vi "ABB Report NoLoad.vi"(10 "Report in":string) -> (2 "Report out":string, 3 "jpg  path":path)   [LabVIEW 2017]
uses:
  ABB global.vi
panel:
  out "Separation of losses":cluster{dbl[], "Best Linear Fit":dbl[]}[](graph)
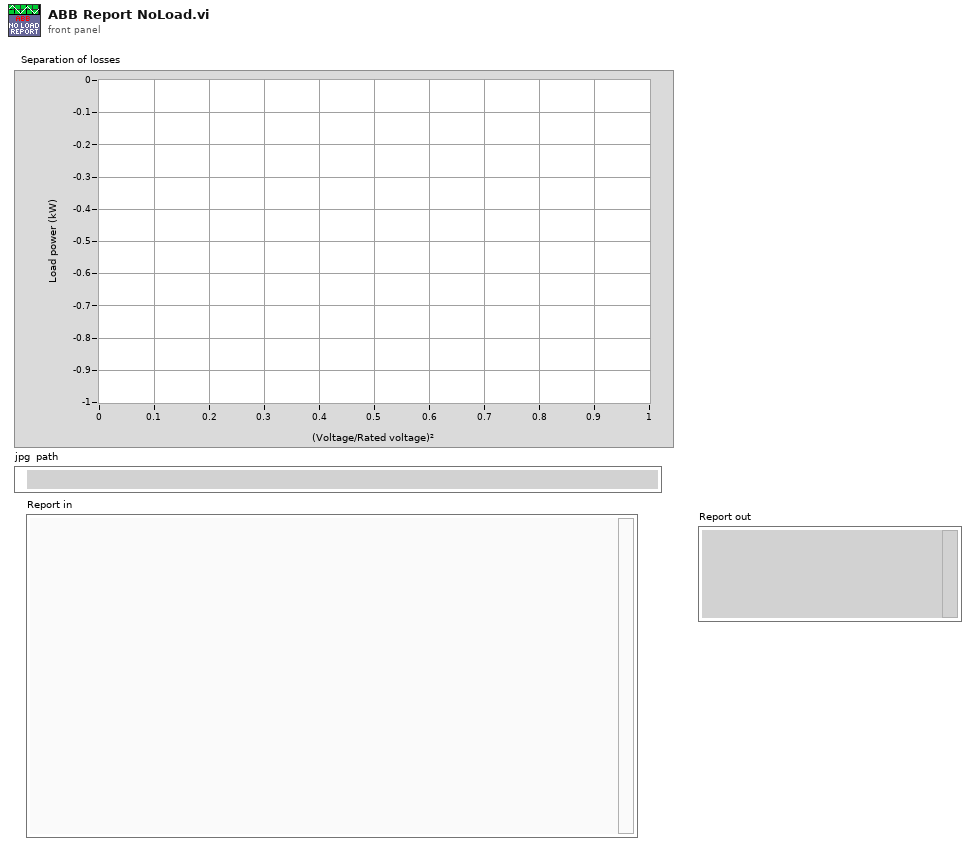
[diagram p1: front panel]
types:
  T1 = cluster{"PCu":dbl, "Pmech":dbl, "PFe":dbl, "Ptot":dbl, "Ambient":dbl, "I1":dbl, "I2":dbl, "I3":dbl, "Wdg Temp":dbl}
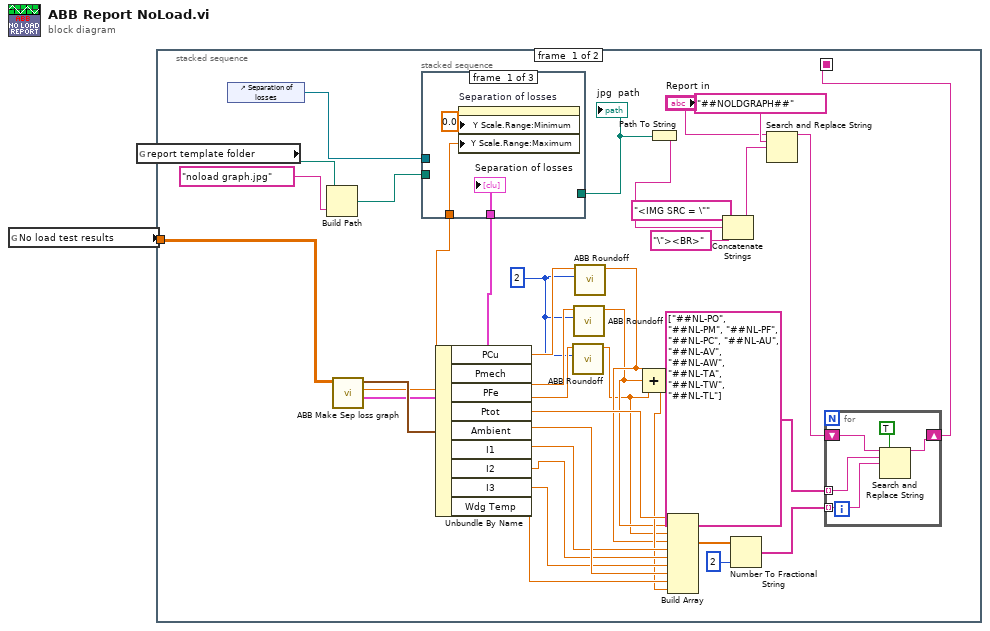
[diagram p0: block diagram]
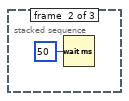
[diagram p2: hidden frame]
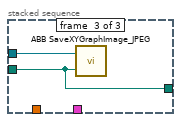
[diagram p3: hidden frame]
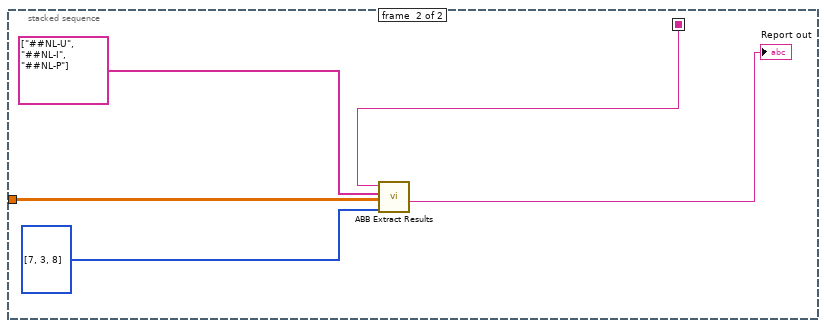
[diagram p4: hidden frame]
diagram:
  n1 = global read "ABB global.vi" "No load test results"() -> (w1:dbl[][])
  n2 = stacked-sequence {
    seq-local: [w24 _] -> [_ w50]
    tunnel: w1 -> [w10 w48]
    frame #0 {
      w2 = 2 ("Precision")
      n3 = global read "ABB global.vi" "report template folder"() -> (w35:path)
      n4 = control-ref of="Separation of losses"() -> (w36:refnum<vi>)
      n5 = Build Path(base path=w35, name or relative path="noload graph.jpg") -> (appended path=w29:path)
      n6 = call "ABB Make Sep loss graph.vi"("Results"=w10) -> ("Sep Loss Graph"=w13:cluster{dbl[], dbl[]}[], "Max Y"=w12:dbl, "Rated V Readings"=w21:T1)  [unwired: 8 in]
      n7 = stacked-sequence {
        tunnel: w36 -> [_ _ w42]
        tunnel: w29 -> [_ _ w41]
        tunnel: w13 -> [w39 _ _]
        tunnel: w12 -> [w37 _ _]
        tunnel: [_ _ w41] -> w11
        frame #0 {
          n8 = property on="Separation of losses" class="XYGraph (strict)"("Y Scale.Range:Minimum"=0.0, "Y Scale.Range:Maximum"=w37) -> ()  [unwired: 2 in, 2 out]
          "Separation of losses" <- w39
        }
        frame #1 {
          n9 = Wait (ms)(milliseconds to wait=u32 50) -> ()  [unwired: 1 out]
        }
        frame #2 {
          n10 = call "ABB SaveXYGraphImage_JPEG.vi"("Path"=w41, "COntrolReference"=w42) -> ()  [unwired: 2 in]
        }
      }
      "jpg  path" <- w11
      n11 = Unbundle By Name(w21) -> ("PCu"=w8:dbl, "Pmech"=w6:dbl, "PFe"=w4:dbl, "Ptot"=w20:dbl, "Ambient"=w19:dbl, "I1"=w18:dbl, "I2"=w17:dbl, "I3"=w16:dbl, "Wdg Temp"=w15:dbl)
      n12 = call "ABB Roundoff.vi"("Precision"=w2, "# in"=w4) -> ("# out"=w3:dbl)  [unwired: 9 in]
      n13 = call "ABB Roundoff.vi"("Precision"=w2, "# in"=w6) -> ("# out"=w5:dbl)  [unwired: 9 in]
      n14 = call "ABB Roundoff.vi"("Precision"=w2, "# in"=w8) -> ("# out"=w7:dbl)  [unwired: 9 in]
      n15 = Compound Arithmetic op=ADD(w7, w5, w3) -> (w14:dbl)
      n16 = Path To String(path=w11) -> (string=w28:string)
      n17 = Build Array(w20, w5, w3, w7, w18, w17, w16, w19, w15, w14) -> (w23:dbl[])
      n18 = Concatenate Strings("<IMG SRC = \"", w28, "\"><BR>" ("string")) -> (w31:string)
      n19 = Number To Fractional String(number=w23, precision (6)=i16 2) -> (F-format string=w22:string[])  [unwired: 2 in]
      n20 = Search and Replace String(input string="Report in", search string="##NOLDGRAPH##", replace string=w31) -> (result string=w25:string)  [unwired: 5 in, 3 out]
      n21 = for {
        tunnel: string[] ["##NL-PO", "##NL-PM", "##NL-PF", "##NL-PC", "##NL-AU", "##NL-AV", "##NL-AW", "##NL-TA", "##NL-TW", "##NL-TL"] -> [w47] mode=indexing
        shift-right: [w45] -> w24
        shift-left: w25 -> [w46]
        tunnel: w22 -> [w44] mode=indexing
        n22 = Search and Replace String(replace all?=TRUE ("replace all? (F)"), input string=w46, search string=w47, replace string=w44) -> (result string=w45:string)  [unwired: 4 in, 3 out]
      }
    }
    frame #1 {
      n23 = call "ABB Extract Results.vi"("Column#"=i32[] [7, 3, 8], "test results"=w48, "ID group"=string[] ["##NL-U", "##NL-I", "##NL-P"], "Report in"=w50) -> ("Report Out"=→"Report out":string)  [unwired: 7 in]
    }
  }
